vi "cm2nm_transform_populate_spot.vi"(1 "NewPointIn":T2, 2 "A - Transformation Matrix":T1, 3 "Previous Session Spot":T2, 4 "C":T1, 5 "B - vector offset":T1, 6 "Spot_ID":string) -> (0 "NewPointOut":T2)   [LabVIEW 2011]
doc: "This is a wrapper routine to call the transform point routine and enter it in the structure for a point."
uses:
  <vilib>/Analysis/Matrix/Datatypes/RealMatrix.ctl
  cm2nm_coordinate_information_v2.ctl
  <vilib>/Analysis/Matrix/NI_Matrix.lvlib
panel:
  # "A(x-c) = y - b"
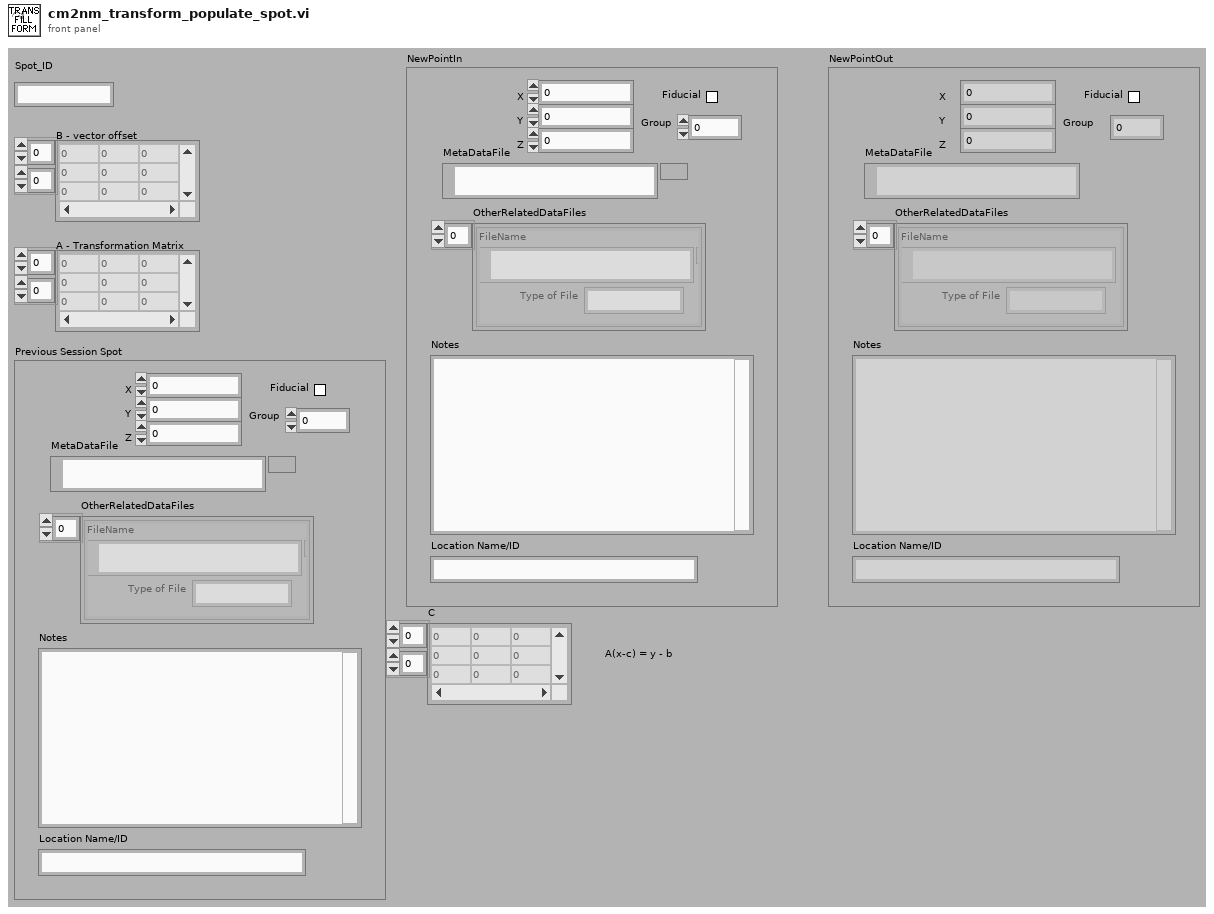
[diagram p1: front panel]
types:
  T1 = typedef "NI_Matrix.lvlib/RealMatrix.ctl" = dbl[][]
  T2 = typedef "cm2nm_coordinate_information_v2.ctl" = cluster{"MetaDataFile":path, "X":dbl, "Y":dbl, "Z":dbl, "Group":i32, "Rotation":dbl[unit], "Fiducial":bool, "Magnification":dbl, "Working_Distance":dbl, "Notes":string, "Location Name/ID":string, "OtherRelatedDataFiles":cluster{"Type of File":string, "FileName":path}[], "Available":bool}
  T3 = cluster{"X1":dbl, "X2":dbl, "Y1":dbl, "Y2":dbl, "Z1":dbl, "Z2":dbl}
  T4 = typedef "Fiducial_pair.ctl" = cluster{"X1":dbl, "X2":dbl, "Y1":dbl, "Y2":dbl, "Z1":dbl, "Z2":dbl}
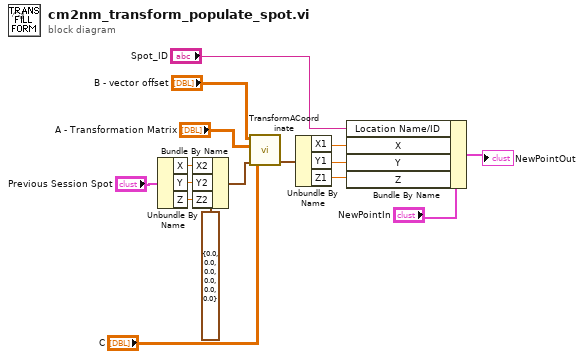
[diagram p0: block diagram]
diagram:
  n1 = Unbundle By Name("Previous Session Spot") -> ("X"=w4:dbl, "Y"=w5:dbl, "Z"=w6:dbl)
  n2 = Bundle By Name(cluster=T3 {"X1"=0.0, "X2"=0.0, "Y1"=0.0, "Y2"=0.0, "Z1"=0.0, "Z2"=0.0} ("Input"), "X2"=w4, "Y2"=w5, "Z2"=w6) -> (w7:T3)
  n3 = call "TransformACoordinate.vi"("Input"=w7, "C"="C", "A"="A - Transformation Matrix", "B"="B - vector offset") -> ("Result"=w8:T4)  [unwired: 1 out]
  n4 = Unbundle By Name(w8) -> ("X1"=w11:dbl, "Y1"=w10:dbl, "Z1"=w9:dbl)
  n5 = Bundle By Name(cluster="NewPointIn", "Location Name/ID"="Spot_ID", "X"=w11, "Y"=w10, "Z"=w9) -> (→"NewPointOut":T2)
